vi "Write Columnname_Alais.vi"(8 "error in (no error)":errorcluster, 10 "Columnname_Alais":string[](array[string]), 11 "SQLite in":refnum<class "SQLite.lvclass">) -> (0 "error out":errorcluster, 3 "SQLite out":refnum<class "SQLite.lvclass">)   [LabVIEW 2017]
uses:
  SQLite.lvclass
  \\vmware-host\Shared Folders/D/Dev/NJAL/OP140/OP140_NJAL_valve_EOL_Test_20210806/Source_Public/DataBase/Top DB/TopDBClass.lvclass
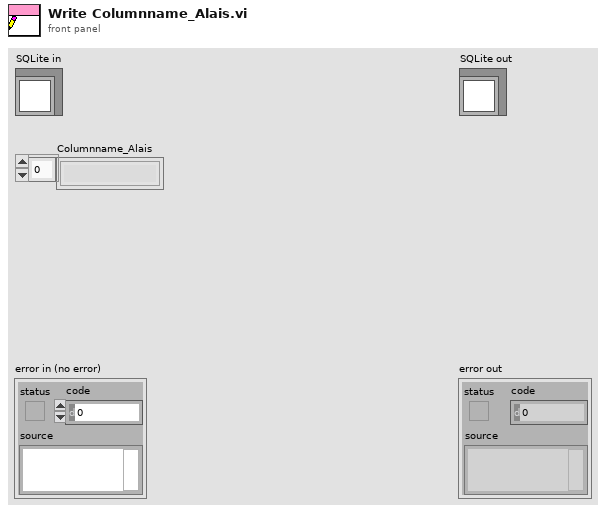
[diagram p1: front panel]
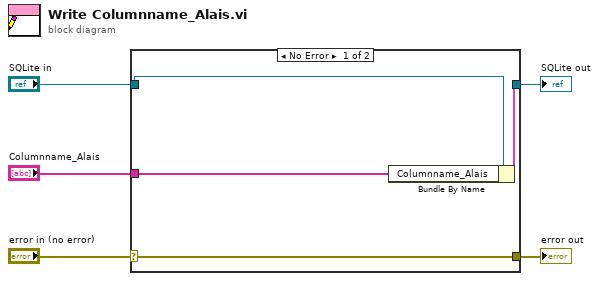
[diagram p0: block diagram]
diagram:
  n1 = case shown="No Error" "error in (no error)" {
    selector: "error in (no error)" -> [w9 w10]
    tunnel: [w9 w10] -> w4
    tunnel: [w7 w11] -> w2
    tunnel: "SQLite in" -> [w8 w11]
    tunnel: "Columnname_Alais" -> [w6 _]
    frame No Error {
      n2 = Bundle By Name(cluster=w8, "Columnname_Alais"=w6) -> (w7:cluster{})
    }
    frame Error {
    }
  }
  "error out" <- w4
  "SQLite out" <- w2
